vi "M Hydro cell.vi"(11 "EV3 in":T1) -> ()   [LabVIEW 2016]
uses:
  <vilib>/NXT/Subs/LVHSConnector.ctl
  <vilib>/NXT/LegoClasses/BrickReference/BrickReference.lvclass
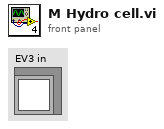
[diagram p1: front panel]
types:
  T1 = typedef "LVHSConnector.ctl" = refnum<class "BrickReference.lvclass">
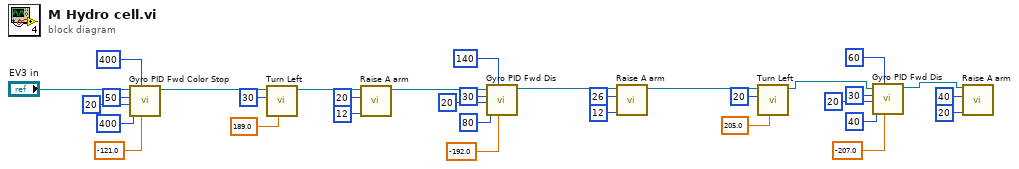
[diagram p0: block diagram]
diagram:
  n1 = call "Gyro PID Fwd Color Stop.vi"("Target angle"=sgl -121.0, "Threshold to Color"=400, "Threshold to slow"=400, "Min. speed"=20, "Max. speed"=50, "EV3 in"="EV3 in") -> ("EV3 out"=w27:T1)  [unwired: 5 in]
  n2 = call "Turn Left.vi"("Turning angle"=sgl 189.0, "Motor B (right)"=i8 30, "EV3 in"=w27) -> ("EV3 out"=w24:T1)  [unwired: 8 in]
  n3 = call "Raise A arm.vi"("Power"=i8 12, "Rotation"=20, "EV3 in"=w24) -> ("EV3 out"=w18:T1)  [unwired: 8 in]
  n4 = call "Gyro PID Fwd Dis.vi"("Target angle"=sgl -192.0, "Threshold to stop"=140, "Threshold to slow"=80, "Min. speed"=20, "Max. speed"=30, "EV3 in"=w18) -> ("EV3 out"=w14:T1)  [unwired: 5 in]
  n5 = call "Raise A arm.vi"("Power"=i8 12, "Rotation"=26, "EV3 in"=w14) -> ("EV3 out"=w11:T1)  [unwired: 8 in]
  n6 = call "Turn Left.vi"("Turning angle"=sgl 205.0, "Motor B (right)"=i8 20, "EV3 in"=w11) -> ("EV3 out"=w2:T1)  [unwired: 8 in]
  n7 = call "Gyro PID Fwd Dis.vi"("Target angle"=sgl -207.0, "Threshold to stop"=60, "Threshold to slow"=40, "Min. speed"=20, "Max. speed"=30, "EV3 in"=w2) -> ("EV3 out"=w1:T1)  [unwired: 5 in]
  n8 = call "Raise A arm.vi"("Power"=i8 20, "Rotation"=40, "EV3 in"=w1) -> ()  [unwired: 8 in, 1 out]
